vi "ATT M2X API.vi"(11 "M2X Action":T1) -> ()   [LabVIEW 2013]
uses:
  Controls/ATT M2X Streams.ctl
  <vilib>/httpClient/POSTBuffer.vi
  <vilib>/httpClient/PUTBuffer.vi
  <vilib>/httpClient/LabVIEWHTTPClient.lvlib
panel:
  out "JSON string":string
  out "URL":string
  out "Response Body":string
  out "Headers":string
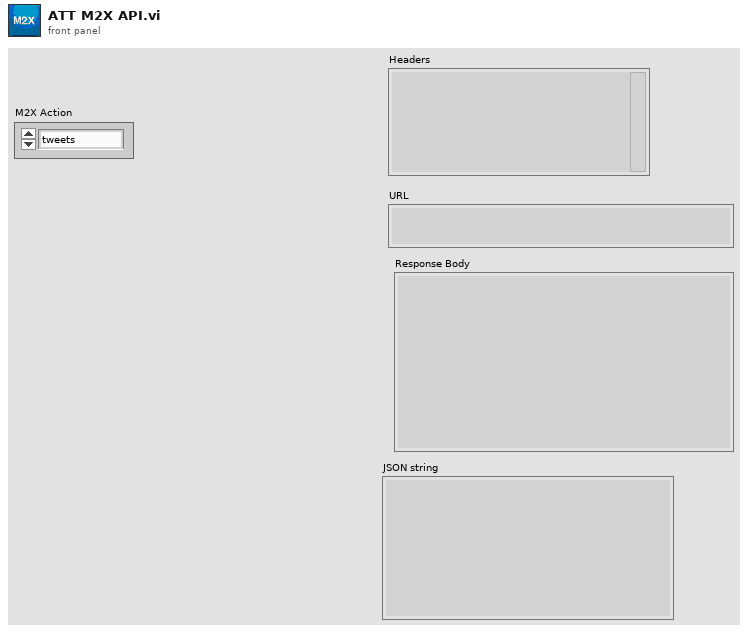
[diagram p1: front panel]
types:
  T1 = typedef "ATT M2X Streams.ctl" = enum16{"tweets", "tweets-make"}
  T2 = typedef "JSON Key List.ctl" = cluster{"X-M2X-KEY":string, "M2X Feed ID":string, "Twitter Access Token":string, "Twitter Access Secret":string, "Twitter Client Token":string, "Twitter Client Secret":string, "NTP Server":string, "Beacons":cluster{"UUID":string, "Major":string, "Minor":string, "BT Address":string}[]}
  T3 = typedef "LabVIEWHTTPClient.lvlib/ClientHandle.ctl" = refnum<k1>
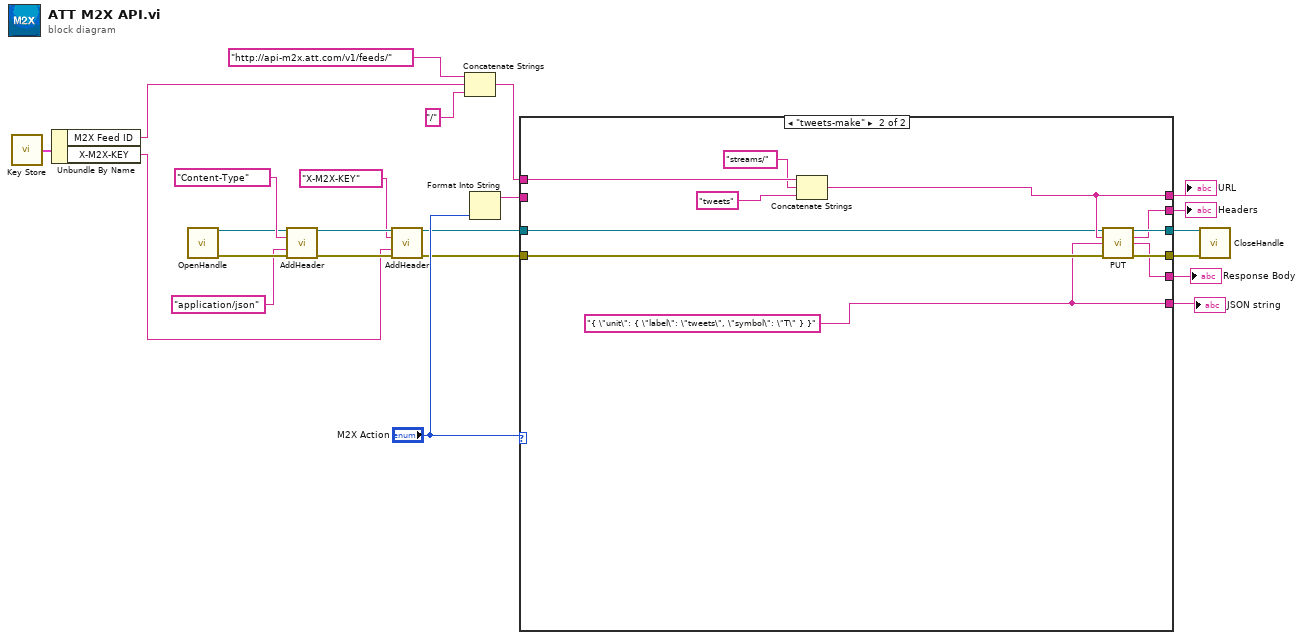
[diagram p0: block diagram]
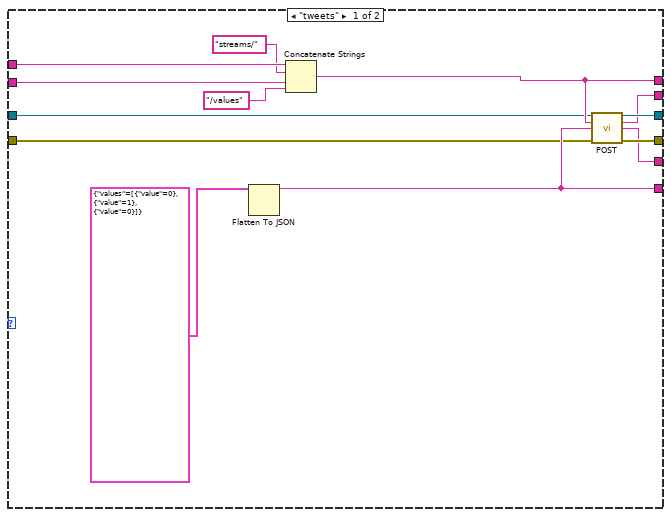
[diagram p2: hidden frame]
diagram:
  n1 = call "Key Store.vi"() -> ("Current Store"=w5:T2)  [unwired: 1 in]
  n2 = Unbundle By Name(w5) -> ("M2X Feed ID"=w4:string, "X-M2X-KEY"=w1:string)
  n3 = call <vilib>:"OpenHandle.vi"() -> ("client handle out"=w19:T3, "error out"=w22:errorcluster)  [unwired: 14 in]
  n4 = call <vilib>:"AddHeader.vi"("client handle"=w19, "header"="Content-Type", "value"="application/json", "error in (no error)"=w22) -> ("client handle out"=w18:T3, "error out"=w17:errorcluster)  [unwired: 10 in]
  n5 = call <vilib>:"AddHeader.vi"("client handle"=w18, "header"="X-M2X-KEY", "value"=w1, "error in (no error)"=w17) -> ("client handle out"=w15:T3, "error out"=w14:errorcluster)  [unwired: 10 in]
  n6 = Concatenate Strings("http://api-m2x.att.com/v1/feeds/" ("url"), w4, "/" ("string")) -> (w2:string)
  n7 = Format Into String("M2X Action") -> (resulting string=w13:string)  [unwired: 3 in, 1 out]
  n8 = case shown="\"tweets-make\"" "M2X Action" {
    tunnel: [w26 w37] -> w7
    tunnel: w15 -> [w24 w39]
    tunnel: [w31 w45] -> w11
    tunnel: w14 -> [w25 w40]
    tunnel: [w30 w44] -> w12
    tunnel: [w27 w41] -> w8
    tunnel: w13 -> [w32 _]
    tunnel: w2 -> [w34 w47]
    tunnel: [w29 w43] -> w10
    tunnel: [w28 w42] -> w9
    frame "tweets" {
      n9 = Flatten To JSON(anything=cluster{"values":cluster{"value":i32}[]} {"values"=[{"value"=0}, {"value"=1}, {"value"=0}]}) -> (JSON string=w26:string)  [unwired: 2 in, 1 out]
      n10 = Concatenate Strings(w34, "streams/" ("string"), w32, "/values" ("string")) -> (w27:string)
      n11 = call-poly <vilib>:"POST.vi"("client handle"=w24, "url"=w27, "buffer"=w26, "error in (no error)"=w25) -> ("client handle out"=w31:T3, "headers"=w29:string, "body"=w28:string, "error out"=w30:errorcluster)  [unwired: 8 in]
    }
    frame "tweets-make" {
      w37 = "{ \"unit\": { \"label\": \"tweets\", \"symbol\": \"T\" } }" ("JSON string")
      n12 = Concatenate Strings(w47, "streams/" ("string"), "tweets" ("string")) -> (w41:string)
      n13 = call-poly <vilib>:"PUT.vi"("client handle"=w39, "url"=w41, "buffer"=w37, "error in (no error)"=w40) -> ("client handle out"=w45:T3, "headers"=w43:string, "body"=w42:string, "error out"=w44:errorcluster)  [unwired: 8 in]
    }
  }
  "Headers" <- w10
  "Response Body" <- w9
  "URL" <- w8
  "JSON string" <- w7
  n14 = call <vilib>:"CloseHandle.vi"("client handle"=w11, "error in (no error)"=w12) -> ()  [unwired: 13 in, 1 out]
